vi "view deploy screen.vi"(8 "error in":errorcluster, 11 "deployment configuration":T1[](array[typedef])) -> (0 "error out":errorcluster)   [LabVIEW 2013, in "PL Framework Configuration Tool.lvlib"]
uses:
  PL Framework Configuration Tool.lvlib
  deployment configuration.ctl
  Framework Configuration Classes/target configuration/PL_Target Configuration.lvclass
  Classes/TBM Configuration Node/deployment configuration.ctl
  Classes/TBM Configuration Node/TBM Configuration Node.lvclass
  Framework Configuration Classes/target configuration/PL_Target Configuration.lvclass/PL_Target Configuration.ctl
  Framework Configuration Classes/target configuration/Read name.vi
  Framework Configuration Classes/target configuration/Read hostname.vi
  Framework Configuration Classes/target configuration/Read OS.vi
  <vilib>/WebDAVClient/Advanced/Put File.vi
  <vilib>/WebDAVClient/NI_WebDAV.lvlib
  <vilib>/FTP/NI_FTP.lvlib
panel:
  in  "password":string
  in  "user":string="admin"
  in  "deploy":bool
  in  "Files to Deploy":i32(listbox)
  in  "targets":i32(listbox)
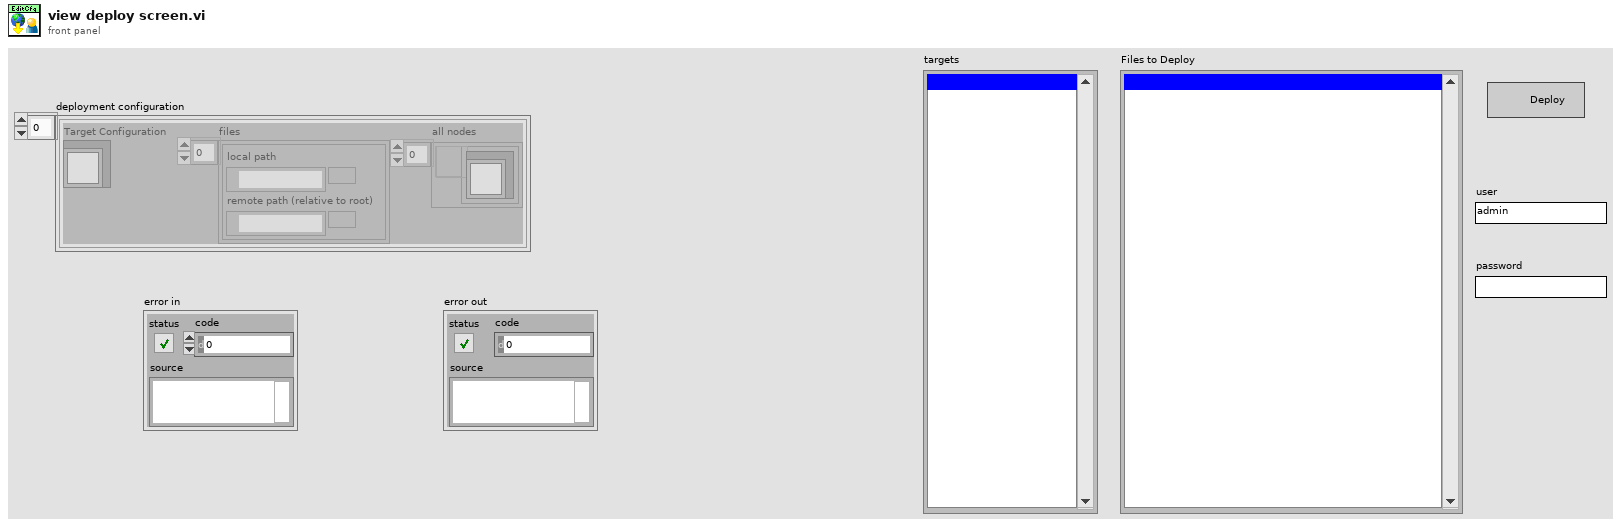
[diagram p1: front panel]
types:
  T1 = typedef "PL Framework Configuration Tool.lvlib/deployment configuration.ctl" = cluster{"Target Configuration":refnum<class "PL_Target Configuration.lvclass">, "files":T2[], "all nodes":refnum<data-value>[]}
  T2 = typedef "PL Framework Configuration Tool.lvlib/TBM Configuration Node.lvclass/deployment configuration.ctl" = cluster{"local path":path, "remote path (relative to root)":path}
  T3 = cluster{"remote path":string, "local path":path, "binary":bool, "path tokens":string[]}
  T4 = typedef "TBM configuration.lvclass/Target Types.ctl" = enum16{"Windows", "Mac", "Linux", "Linux RT ARM", "VxWorks", "Pharlap", "Other", "Linux RT x64"}
  T5 = typedef "NI_WebDAV.lvlib/SessionHandle.ctl" = refnum<k1>
  T6 = typedef "NI_FTP.lvlib/FTP Session.ctl" = refnum<k5>
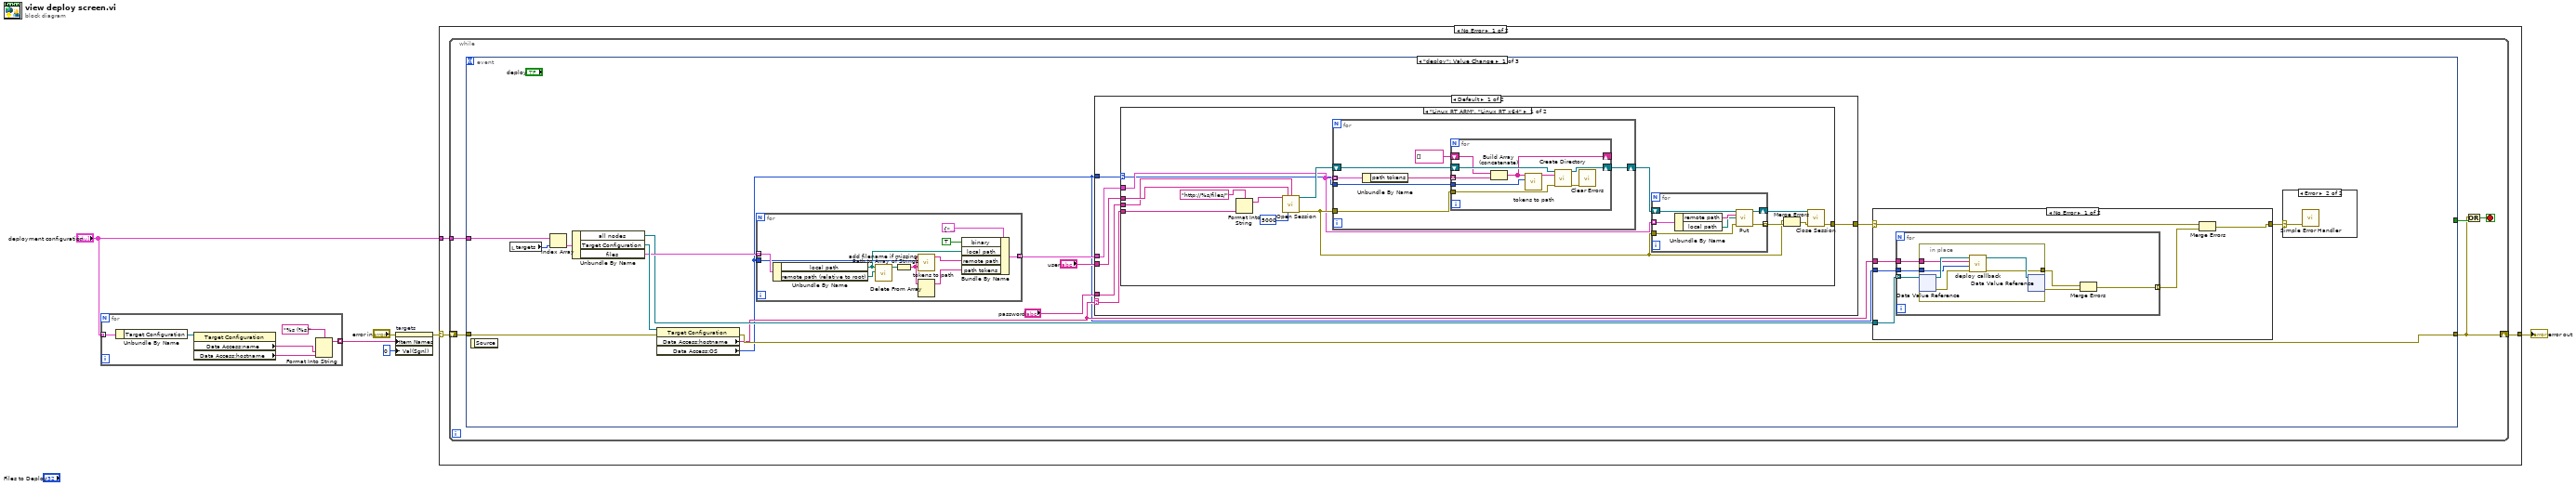
[diagram p0: block diagram]
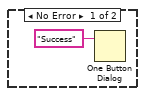
[diagram p2: hidden frame]
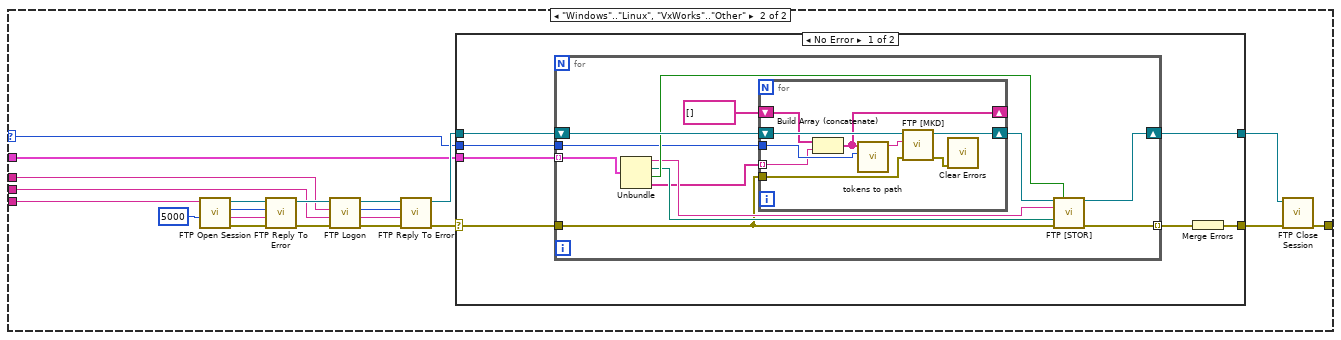
[diagram p3: hidden frame]
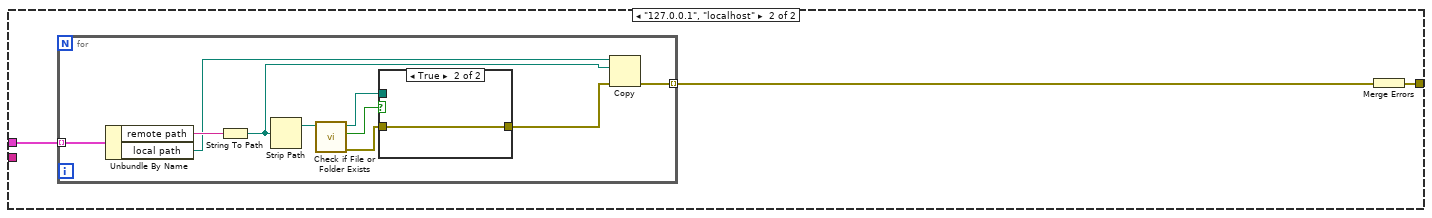
[diagram p5: hidden frame]
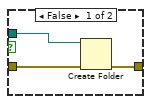
[diagram p6: hidden frame]
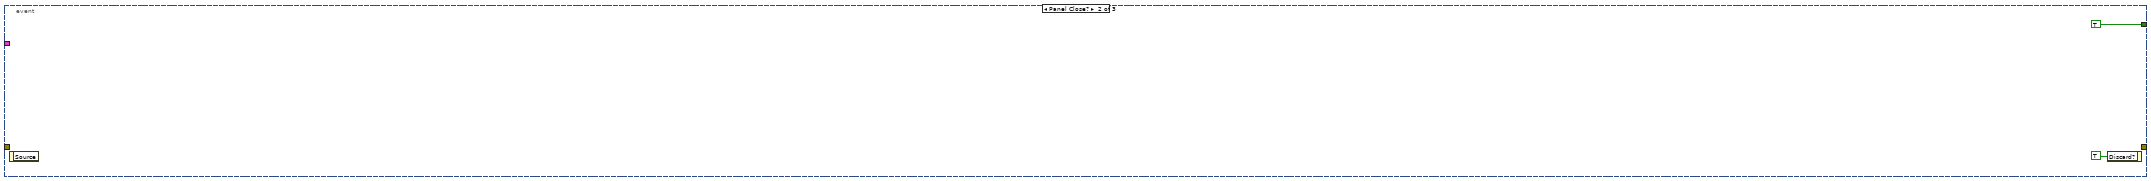
[diagram p8: hidden frame]
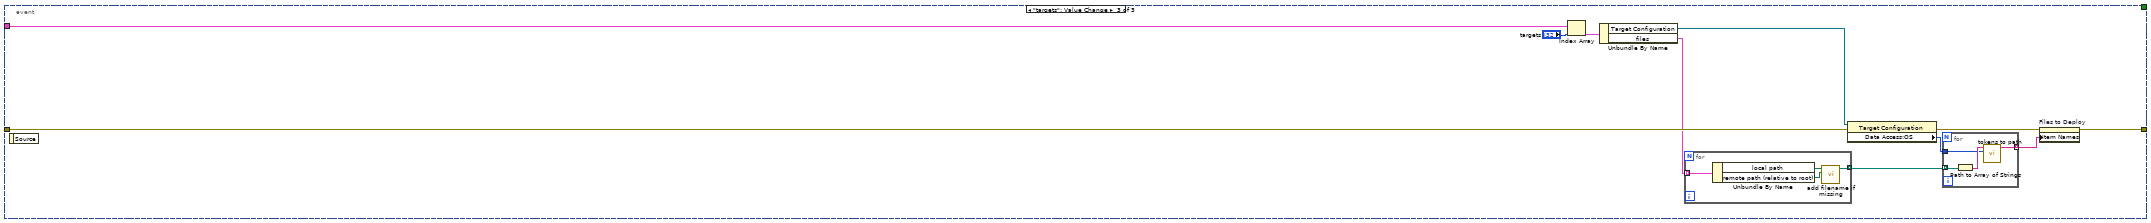
[diagram p9: hidden frame]
diagram:
  n1 = for {
    tunnel: "deployment configuration" -> [w12] mode=indexing
    tunnel: [w7] -> w6 mode=indexing
    n2 = Unbundle By Name(w12) -> ("Target Configuration"=w11:refnum<class "PL_Target Configuration.lvclass">)
    n3 = property class="Target Configuration"(reference=w11) -> ("Data Access:name"=w10:string, "Data Access:hostname"=w9:string)  [unwired: 1 in, 2 out]
    n4 = Format Into String(format string="%s (%s)", w10, w9) -> (resulting string=w7:string)  [unwired: 2 in, 1 out]
  }
  n5 = property on="targets" class="LstBox (strict)"(error in="error in", "Item Names"=w6, "Val(Sgnl)"=0 ("Value (Signaling)")) -> (error out=w3:errorcluster)  [unwired: 1 in, 1 out]
  n6 = case shown="No Error" w3 {
    selector: w3 -> [w15 w201]
    tunnel: [w14 w201] -> w2
    tunnel: "deployment configuration" -> [w13 _]
    frame No Error {
      n7 = while {
        shift-right: [w17] -> w14
        shift-left: w15 -> [w19]
        tunnel: w13 -> [w16]
        stop <- w18 stop-if-true
        n8 = event shown="[0] \"deploy\": Value Change" {
          selector: _ -> [_ _ _]
          dyn-events: _ -> [_ _ _]
          timeout: _ -> [_ _ _]
          tunnel: [_ TRUE ("Cancel Button") _] -> w20
          tunnel: w19 -> [w30 _ w189]
          tunnel: [w29 _ w187] -> w17
          tunnel: w16 -> [w33 _ w192]
          event "deploy": Value Change {
            n9 = event-data() -> ()  [unwired: 1 in, 1 out]
            n10 = local read "targets"() -> (w32:i32)
            n11 = Index Array(array=w33, index=w32) -> (element=w35:T1)
            n12 = Unbundle By Name(w35) -> ("all nodes"=w24:refnum<data-value>[], "Target Configuration"=w34:refnum<class "PL_Target Configuration.lvclass">, "files"=w31:T2[])
            n13 = property class="Target Configuration"(reference=w34, error in=w30) -> (error out=w29:errorcluster, "Data Access:hostname"=w22:string, "Data Access:OS"=w21:T4)  [unwired: 1 out]
            n14 = for {
              tunnel: w31 -> [w179] mode=indexing
              tunnel: [w176] -> w28 mode=indexing
              tunnel: w21 -> [w173]
              n15 = Unbundle By Name(w179) -> ("local path"=w170:path, "remote path (relative to root)"=w171:path)
              n16 = call "add filename if missing.vi"("remote path (relative to root)"=w171, "local path"=w170) -> ("appended path"=w169:path)  [unwired: 9 in]
              n17 = Path to Array of Strings(0:w169) -> (2:w174:string[])  [unwired: 1 out]
              n18 = call "tokens to path.vi"("Data Access:OS"=w173, "array of strings"=w174) -> ("String"=w175:string)  [unwired: 9 in]
              n19 = Delete From Array(array=w174) -> (array with subset deleted=w172:string[])  [unwired: 2 in, 1 out]
              n20 = Bundle By Name(cluster=T3 {"remote path"="", "local path"=path "", "binary"=FALSE, "path tokens"=[]} ("transfer spec"), "binary"=TRUE, "local path"=w170, "remote path"=w175, "path tokens"=w172) -> (w176:T3)
            }
            n21 = case shown="Default" w22 {
              selector: w22 -> [w38 _]
              tunnel: w28 -> [w43 w135]
              tunnel: w21 -> [w42 _]
              tunnel: "user" -> [w41 _]
              tunnel: "password" -> [w40 _]
              tunnel: [w39 w133] -> w25
              frame Default {
                n22 = case shown="\"Linux RT ARM\", \"Linux RT x64\"" w42 {
                  selector: w42 -> [w45 w83]
                  tunnel: w43 -> [w46 w84]
                  tunnel: w38 -> [w51 w92]
                  tunnel: [w56 w85] -> w39
                  tunnel: w41 -> [w58 w91]
                  tunnel: w40 -> [w57 w90]
                  frame "Linux RT ARM", "Linux RT x64" {
                    n23 = Format Into String(format string="http://%s/files/", w51) -> (resulting string=w52:string)  [unwired: 2 in, 1 out]
                    n24 = call <vilib>:"Open Session.vi"("host uri prefix"=w52, "username"=w58, "password"=w57, "timeout ms"=5000) -> ("session handle out"=w49:T5, "error out"=w47:errorcluster)  [unwired: 10 in]
                    n25 = for {
                      tunnel: w47 -> [w62]
                      shift-right: [w63] -> w48
                      shift-left: w49 -> [w64]
                      tunnel: w46 -> [w65] mode=indexing
                      tunnel: w45 -> [w61]
                      n26 = Unbundle By Name(w65) -> ("path tokens"=w60:string[])
                      n27 = for {
                        tunnel: w62 -> [w72]
                        tunnel: w61 -> [w70]
                        tunnel: w60 -> [w67] mode=indexing
                        shift-right: [w66] -> _
                        shift-left: string[] [] ("path tokens") -> [w68]
                        shift-right: [w73] -> w63
                        shift-left: w64 -> [w74]
                        n28 = Build Array (concatenate)(w68, w67) -> (w66:string[])
                        n29 = call "tokens to path.vi"("Data Access:OS"=w70, "array of strings"=w66) -> ("String"=w69:string)  [unwired: 9 in]
                        n30 = call <vilib>:"Create Directory.vi"("session handle"=w74, "relative uri"=w69, "error in (no error)"=w72) -> ("session handle out"=w73:T5, "error out"=w71:errorcluster)  [unwired: 11 in]
                        n31 = call <vilib>:"Clear Errors.vi"("error in (no error)"=w71) -> ()  [unwired: 6 in, 1 out]
                      }
                    }
                    n32 = for {
                      tunnel: w47 -> [w81]
                      tunnel: [w80] -> w54 mode=indexing
                      shift-right: [w78] -> w53
                      shift-left: w48 -> [w79]
                      tunnel: w46 -> [w77] mode=indexing
                      n33 = Unbundle By Name(w77) -> ("remote path"=w76:string, "local path"=w75:path)
                      n34 = call-poly <vilib>:"Put.vi"("session handle"=w79, "relative uri"=w76, "local file path"=w75, "error in (no error)"=w81) -> ("session handle out"=w78:T5, "error out"=w80:errorcluster)  [unwired: 9 in, 1 out]
                    }
                    n35 = Merge Errors(w47, w54) -> (w55:errorcluster)
                    n36 = call <vilib>:"Close Session.vi"("session handle"=w53, "error in (no error)"=w55) -> ("error out"=w56:errorcluster)  [unwired: 13 in]
                  }
                  frame "Windows".."Linux", "VxWorks".."Other" {
                    n37 = call <vilib>:"FTP Open Session.vi"("timeout ms (60000)"=5000, "address"=w92) -> ("error out"=w93:errorcluster, "reply string"=w96:string, "reply code"=w95:i32, "ftp session"=w94:T6)  [unwired: 2 in, 4 out]
                    n38 = call <vilib>:"FTP Reply To Error.vi"("error in (no error)"=w93, "reply string in"=w96, "reply code in"=w95, "ftp session"=w94) -> ("error out"=w98:errorcluster, "ftp session out"=w97:T6)  [unwired: 2 out]
                    n39 = call <vilib>:"FTP Logon.vi"("error in (no error)"=w98, "password"=w90, "user"=w91, "ftp session"=w97) -> ("error out"=w99:errorcluster, "reply string"=w102:string, "reply code"=w101:i32, "ftp session out"=w100:T6)  [unwired: 4 out]
                    n40 = call <vilib>:"FTP Reply To Error.vi"("error in (no error)"=w99, "reply string in"=w102, "reply code in"=w101, "ftp session"=w100) -> ("error out"=w87:errorcluster, "ftp session out"=w89:T6)  [unwired: 2 out]
                    n41 = case shown="No Error" w87 {
                      selector: w87 -> [w107 w132]
                      tunnel: w89 -> [w109 w131]
                      tunnel: [w108 w131] -> w88
                      tunnel: [w105 w132] -> w86
                      tunnel: w84 -> [w104 _]
                      tunnel: w83 -> [w103 _]
                      frame No Error {
                        n42 = for {
                          shift-right: [w119] -> w108
                          shift-left: w109 -> [w121]
                          tunnel: w107 -> [w110]
                          tunnel: [w120] -> w106 mode=indexing
                          tunnel: w104 -> [w117] mode=indexing
                          tunnel: w103 -> [w112]
                          n43 = Unbundle(w117) -> ("remote path"=w114:string, "local path"=w115:path, "binary"=w116:bool, "path tokens"=w113:string[])
                          n44 = for {
                            tunnel: w110 -> [w128]
                            tunnel: w113 -> [w124] mode=indexing
                            tunnel: w112 -> [w127]
                            shift-right: [w129] -> w118
                            shift-left: w121 -> [w130]
                            shift-right: [w123] -> _
                            shift-left: string[] [] ("path tokens") -> [w125]
                            n45 = Build Array (concatenate)(w125, w124) -> (w123:string[])
                            n46 = call "tokens to path.vi"("Data Access:OS"=w127, "array of strings"=w123) -> ("String"=w126:string)  [unwired: 9 in]
                            n47 = call <vilib>:"FTP [MKD].vi"("error in (no error)"=w128, "directory path"=w126, "ftp session"=w130) -> ("error out"=w122:errorcluster, "ftp session out"=w129:T6)  [unwired: 5 in, 2 out]
                            n48 = call <vilib>:"Clear Errors.vi"("error in (no error)"=w122) -> ()  [unwired: 6 in, 1 out]
                          }
                          n49 = call <vilib>:"FTP [STOR].vi"("ftp session"=w118, "binary (F)"=w116, "remote path"=w114, "local path (<NAP>)"=w115, "error in (no error)"=w110) -> ("ftp session out"=w119:T6, "error out"=w120:errorcluster)  [unwired: 1 in, 8 out]
                        }
                        n50 = Merge Errors(w106) -> (w105:errorcluster)
                      }
                      frame Error {
                      }
                    }
                    n51 = call <vilib>:"FTP Close Session.vi"("error in (no error)"=w86, "ftp session"=w88) -> ("error out"=w85:errorcluster)  [unwired: 9 out]
                  }
                }
              }
              frame "127.0.0.1", "localhost" {
                n52 = for {
                  tunnel: [w144] -> w134 mode=indexing
                  tunnel: w135 -> [w145] mode=indexing
                  n53 = Unbundle By Name(w145) -> ("remote path"=w143:string, "local path"=w137:path)
                  n54 = String To Path(string=w143) -> (path=w136:path)
                  n55 = Strip Path(path=w136) -> (stripped path=w141:path)  [unwired: 1 out]
                  n56 = call <vilib>:"Check if File or Folder Exists.vi"("path"=w141) -> ("error out"=w139:errorcluster, "file or folder exists?"=w140:bool, "dup path"=w142:path)  [unwired: 8 in]
                  n57 = case shown="True" w140 {
                    tunnel: w142 -> [w148 _]
                    tunnel: w139 -> [w147 w149]
                    tunnel: [w146 w149] -> w138
                    frame False {
                      n58 = Create Folder(path (use dialog)=w148, error in=w147) -> (error out=w146:errorcluster)  [unwired: 1 in, 2 out]
                    }
                    frame True {
                    }
                  }
                  n59 = Copy(8:w138, 10:w136, 11:w137) -> (0:w144:errorcluster)  [unwired: 2 in, 2 out]
                }
                n60 = Merge Errors(w134) -> (w133:errorcluster)
              }
            }
            n61 = case shown="No Error" w25 {
              selector: w25 -> [w152 w168]
              tunnel: w24 -> [w155 _]
              tunnel: [w154 w168] -> w23
              tunnel: w22 -> [w151 _]
              tunnel: w21 -> [w150 _]
              frame No Error {
                n62 = for {
                  tunnel: w155 -> [w161] mode=indexing
                  tunnel: [w160] -> w153 mode=indexing
                  tunnel: w151 -> [w157]
                  tunnel: w150 -> [w156]
                  n63 = in-place {
                    in-place-border: [w165] -> w158
                    in-place-border: w157 -> [w163]
                    in-place-border: w156 -> [w162]
                    n64 = in-place-dvr #1(w161) -> (w167:refnum<class "TBM Configuration Node.lvclass">, w164:errorcluster)
                    n65 = call-dynamic "deploy callback.vi"("error in"=w164, "Target Types"=w162, "IP Address"=w163, "TBM Configuration Node in"=w167) -> ("error out"=w165:errorcluster, "TBM Configuration Node out"=w166:refnum<class "TBM Configuration Node.lvclass">)  [unwired: 6 in]
                    n66 = in-place-dvr #1(w166) -> (w159:errorcluster)  [unwired: 1 out]
                  }
                  n67 = Merge Errors(w158, w159) -> (w160:errorcluster)
                }
                n68 = Merge Errors(w152, w153) -> (w154:errorcluster)
              }
              frame Error {
              }
            }
            n69 = case shown="Error" w23 {
              selector: w23 -> [_ w37]
              frame No Error {
                n70 = One Button Dialog(message="Success") -> ()  [unwired: 1 in, 1 out]
              }
              frame Error {
                n71 = call <vilib>:"Simple Error Handler.vi"("error in (no error)"=w37) -> ()  [unwired: 4 in, 5 out]
              }
            }
          }
          event Panel Close? {
            n72 = event-data() -> ()  [unwired: 1 in, 1 out]
            n73 = event-data("Discard?"=TRUE) -> ()  [unwired: 1 in, 1 out]
          }
          event "targets": Value Change {
            n74 = event-data() -> ()  [unwired: 1 in, 1 out]
            n75 = Index Array(array=w192, index="targets") -> (element=w190:T1)
            n76 = Unbundle By Name(w190) -> ("Target Configuration"=w185:refnum<class "PL_Target Configuration.lvclass">, "files"=w188:T2[])
            n77 = for {
              tunnel: w188 -> [w200] mode=indexing
              tunnel: [w197] -> w184 mode=indexing
              n78 = Unbundle By Name(w200) -> ("local path"=w199:path, "remote path (relative to root)"=w198:path)
              n79 = call "add filename if missing.vi"("remote path (relative to root)"=w198, "local path"=w199) -> ("appended path"=w197:path)  [unwired: 9 in]
            }
            n80 = property class="Target Configuration"(reference=w185, error in=w189) -> (error out=w186:errorcluster, "Data Access:OS"=w183:T4)  [unwired: 1 out]
            n81 = for {
              tunnel: w184 -> [w195] mode=indexing
              tunnel: w183 -> [w194]
              tunnel: [w193] -> w182 mode=indexing
              n82 = Path to Array of Strings(0:w195) -> (2:w196:string[])  [unwired: 1 out]
              n83 = call "tokens to path.vi"("Data Access:OS"=w194, "array of strings"=w196) -> ("String"=w193:string)  [unwired: 9 in]
            }
            n84 = property on="Files to Deploy" class="LstBox (strict)"(error in=w186, "Item Names"=w182) -> (error out=w187:errorcluster)  [unwired: 1 in, 1 out]
          }
        }
        n85 = Or(x=w17, y=w20) -> (x .or. y?=w18:bool)
      }
    }
    frame Error {
    }
  }
  "error out" <- w2
